vi "Extract.vi"(8 "error in (no error)":errorcluster, 11 "Vision in":refnum<class "Vision.lvclass">) -> (0 "error out":errorcluster, 3 "Vision out":refnum<class "Vision.lvclass">)   [LabVIEW 2019, in "Vision.lvlib" / "Vision.lvclass"]
uses:
  Vision.lvclass
  Vision.lvclass/Vision.ctl
  <vilib>/vision/NI_Vision_Development_Module.lvlib
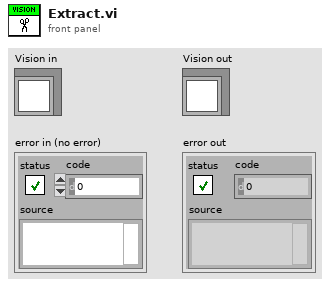
[diagram p1: front panel]
types:
  T1 = cluster{"Contour Type":u32, "ROI Type":u32, "Points":i32[]}[]
  T2 = typedef "IMAQ Image.ctl" = refnum<image>
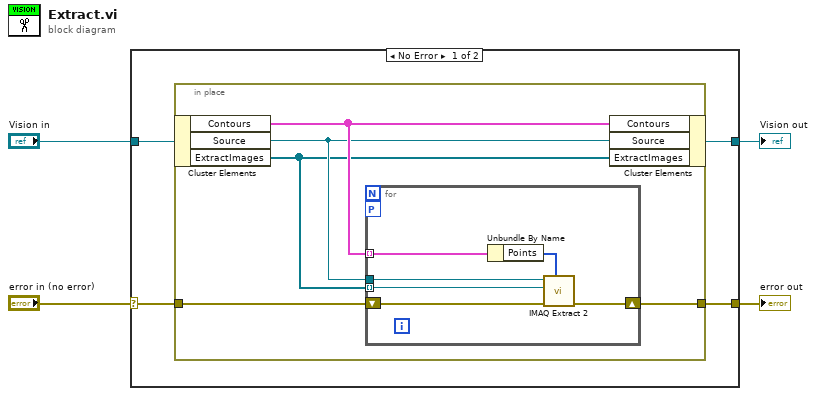
[diagram p0: block diagram]
diagram:
  n1 = case shown="No Error" "error in (no error)" {
    selector: "error in (no error)" -> [w6 w21]
    tunnel: [w5 w21] -> w3
    tunnel: [w7 w20] -> w1
    tunnel: "Vision in" -> [w8 w20]
    frame No Error {
      n2 = in-place {
        in-place-border: w6 -> [w13]
        in-place-border: [w12] -> w5
        n3 = in-place-cluster #1(w8) -> ("Contours"=w11:T1, "Source"=w10:T2, "ExtractImages"=w9:T2[])
        n4 = for {
          tunnel: w11 -> [w19] mode=indexing
          shift-right: [w17] -> w12
          shift-left: w13 -> [w15]
          tunnel: w9 -> [w16] mode=indexing
          tunnel: w10 -> [w14]
          workers-P: _ -> [_]
          n5 = Unbundle By Name(w19) -> ("Points"=w18:i32[])
          n6 = call "IMAQ Extract 2"("Optional Rectangle"=w18, "error in (no error)"=w15, "Image Dst"=w16, "Image Src"=w14) -> ("error out"=w17:errorcluster)  [unwired: 6 in, 1 out]
        }
        n7 = in-place-cluster #1("Contours"=w11, "Source"=w10, "ExtractImages"=w9) -> (w7:refnum<class "Vision.lvclass">)
      }
    }
    frame Error {
    }
  }
  "error out" <- w3
  "Vision out" <- w1
